vi "WriteWiringToMap.vi"(8 "error in (no error)":errorcluster, 9 "Map in":T12, 10 "Working Current":T1, 11 "Group":T2) -> (0 "error out":errorcluster, 1 "Map out":T12, 3 "Group out":T2)   [LabVIEW 2017, in "McsaAnalysisLowRate.lvlib"]
uses:
  <vilib>/addons/InsightCM/Devices/Shared/Mcsa/McsaAnalysisLowRate/McsaAnalysisLowRate.lvlib
  <vilib>/addons/PointValueMap/controls/PointMap.ctl
  <vilib>/addons/InsightCM/Devices/Shared/Mcsa/McsaAnalysisLowRate/controls/Group.ctl
  <vilib>/addons/InsightCM/Utilities/Analysis/MCSA/controls/McsaChannel.ctl
  <vilib>/addons/InsightCM/Utilities/Analysis/Shared/controls/Feature.ctl
  <vilib>/addons/InsightCM/Utilities/Analysis/Shared/controls/AmplitudeScale.ctl
  <vilib>/addons/InsightCM/MessageBus/Base/controls/KeyValuePair.ctl
  <vilib>/addons/InsightCM/Utilities/Analysis/MCSA/controls/McsaChannelPhasor.ctl
  <vilib>/addons/InsightCM/Utilities/Analysis/MCSA/controls/McsaMotor.ctl
  <vilib>/addons/InsightCM/Utilities/Analysis/MCSA/controls/MotorCalculationCache.ctl
  <vilib>/addons/Electrical Power/Basic/Measurement/subVIs/basic_Power Value.ctl
  <vilib>/addons/InsightCM/Utilities/Analysis/MCSA/controls/TorqueLoadEfficiency.ctl
  <vilib>/addons/InsightCM/Utilities/Analysis/MCSA/controls/WorkingCurrent.ctl
  <vilib>/addons/InsightCM/Utilities/MCSA/McsaUtilities.lvlib
  <vilib>/addons/PointValueMap/PointValueMap.lvlib
  <vilib>/addons/InsightCM/Utilities/Analysis/Shared/AnalysisHelper.lvlib
  <vilib>/addons/InsightCM/Utilities/Analysis/MCSA/McsaAnalysisFunctions.lvlib
  <vilib>/addons/Electrical Power/Basic/NI_EP_Basic.lvlib
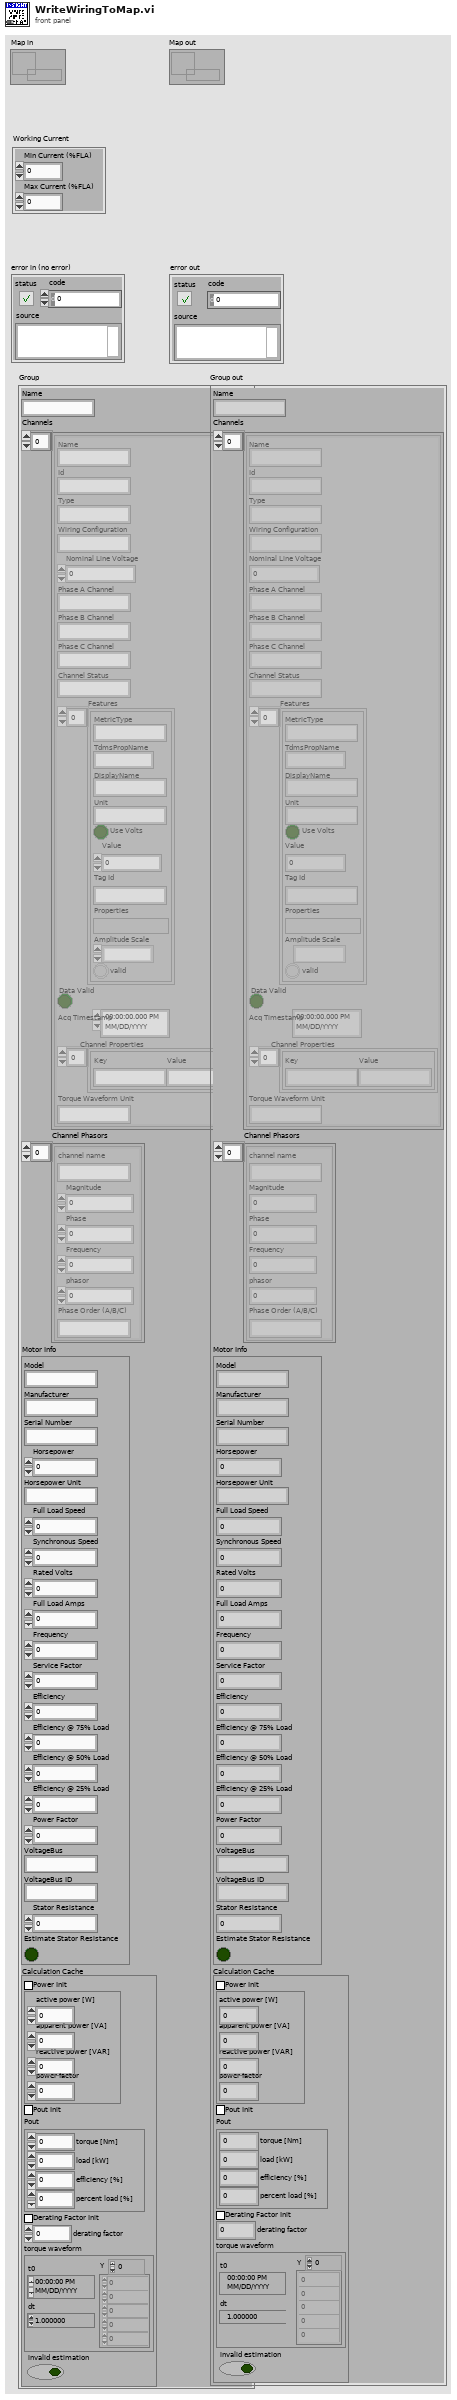
[diagram p1: front panel]
types:
  T1 = typedef "McsaAnalysisFunctions.lvlib/WorkingCurrent.ctl" = cluster{"Min Current (%FLA)":dbl, "Max Current (%FLA)":dbl}
  T2 = typedef "McsaAnalysisLowRate.lvlib/Group.ctl" = cluster{"Name":string, "Channels":T3[], "Channel Phasors":T7[], "Motor Info":T8, "Calculation Cache":T9}
  T3 = typedef "McsaAnalysisFunctions.lvlib/McsaChannel.ctl" = cluster{"Name":string, "Id":string, "Type":string, "Wiring Configuration":string, "Nominal Line Voltage":dbl, "Phase A Channel":string, "Phase B Channel":string, "Phase C Channel":string, "Channel Status":string, "Features":T4[], "Data Valid":bool, "Acq Timestamp":timestamp, "Channel Properties":T6[], "Torque Waveform Unit":string}
  T4 = typedef "AnalysisHelper.lvlib/Feature.ctl" = cluster{"MetricType":string, "TdmsPropName":string, "DisplayName":string, "Unit":string, "Use Volts":bool, "Value":dbl, "Tag Id":string, "Properties":variant, "Amplitude Scale":T5, "valid":bool}
  T5 = typedef "AnalysisHelper.lvlib/AmplitudeScale.ctl" = enum16{"rms", "peak", "pk-pk"}
  T6 = typedef "KeyValuePair.ctl" = cluster{"Key":string, "Value":string}
  T7 = typedef "McsaAnalysisFunctions.lvlib/McsaChannelPhasor.ctl" = cluster{"channel name":string, "Magnitude":dbl, "Phase":dbl, "Frequency":dbl, "phasor":cdb, "Phase Order (A/B/C)":string}
  T8 = typedef "McsaAnalysisFunctions.lvlib/McsaMotor.ctl" = cluster{"Model":string, "Manufacturer":string, "Serial Number":string, "Horsepower":dbl, "Horsepower Unit":string, "Full Load Speed":dbl, "Synchronous Speed":dbl, "Rated Volts":dbl, "Full Load Amps":dbl, "Frequency":dbl, "Service Factor":dbl, "Efficiency":dbl, "Efficiency @ 75% Load":dbl, "Efficiency @ 50% Load":dbl, "Efficiency @ 25% Load":dbl, "Power Factor":dbl, "VoltageBus":string, "VoltageBus ID":string, "Stator Resistance":dbl, "Estimate Stator Resistance":bool}
  T9 = typedef "McsaAnalysisFunctions.lvlib/MotorCalculationCache.ctl" = cluster{"Power Init":bool, "power value":T10, "Pout Init":bool, "Pout":T11, "Derating Factor Init":bool, "derating factor":sgl, "torque waveform":waveform(dbl), "invalid estimation":bool}
  T10 = typedef "NI_EP_Basic.lvlib/basic_Power Value.ctl" = cluster{"active power [W]":dbl, "apparent power [VA]":dbl, "reactive power [VAR]":dbl, "power factor":dbl}
  T11 = typedef "McsaAnalysisFunctions.lvlib/TorqueLoadEfficiency.ctl" = cluster{"torque [Nm]":dbl, "load [kW]":dbl, "efficiency [%]":dbl, "percent load [%]":dbl}
  T12 = typedef "PointValueMap.lvlib/PointMap.ctl" = refnum<data-value>
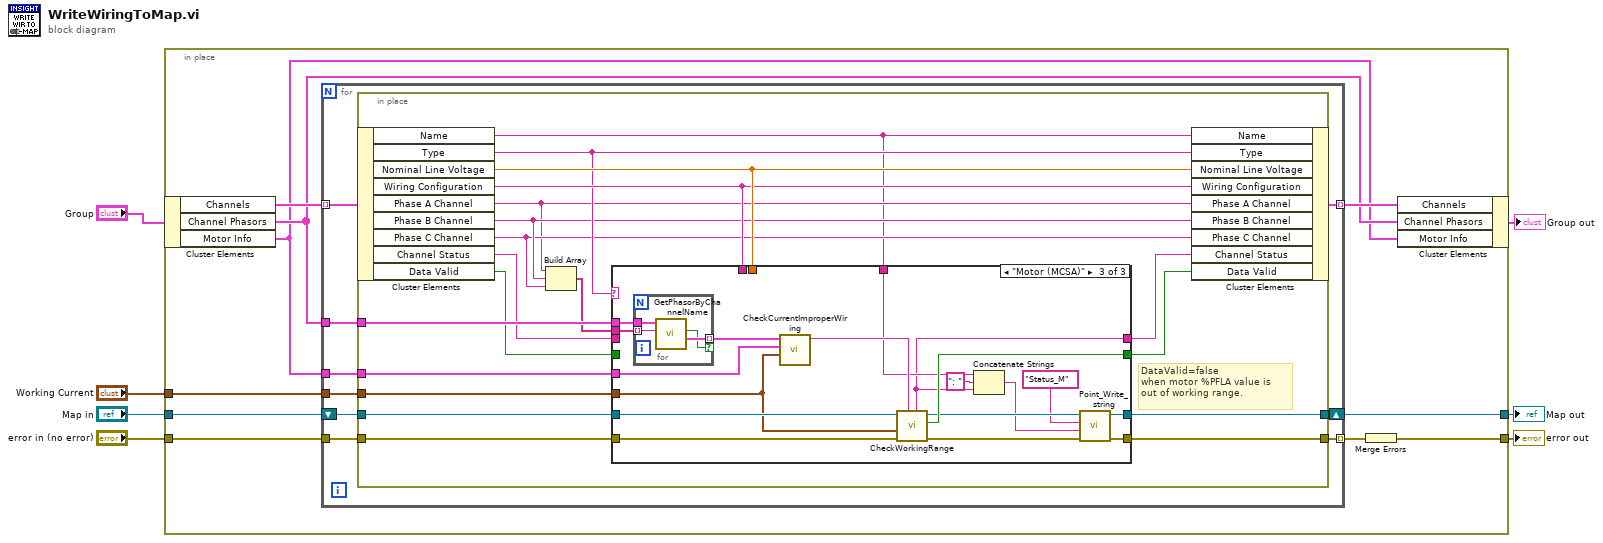
[diagram p0: block diagram]
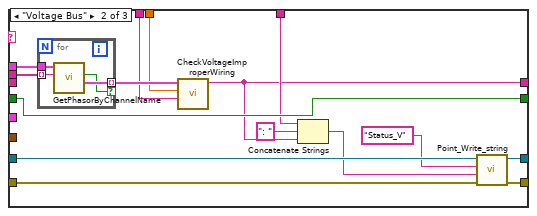
[diagram p3: hidden frame]
diagram:
  n1 = in-place {
    in-place-border: "Map in" -> [w17]
    in-place-border: "error in (no error)" -> [w16]
    in-place-border: [w10] -> w7
    in-place-border: [w9] -> w4
    in-place-border: "Working Current" -> [w11]
    n2 = in-place-cluster #1("Group") -> ("Channels"=w14:T3[], "Channel Phasors"=w12:T7[], "Motor Info"=w8:T8)
    n3 = for {
      tunnel: w14 -> [w21] mode=indexing
      tunnel: w16 -> [w25]
      tunnel: [w24] -> w15 mode=indexing
      shift-right: [w23] -> w9
      shift-left: w17 -> [w26]
      tunnel: [w22] -> w13 mode=indexing
      tunnel: w12 -> [w20]
      tunnel: w11 -> [w19]
      tunnel: w8 -> [w18]
      n4 = in-place {
        in-place-border: w26 -> [w45]
        in-place-border: w25 -> [w44]
        in-place-border: [w38] -> w24
        in-place-border: [w43] -> w23
        in-place-border: w20 -> [w42]
        in-place-border: w19 -> [w36]
        in-place-border: w18 -> [w27]
        # "DataValid=false\nwhen motor %PFLA value is \nout of working range."
        n5 = in-place-cluster #2(w21) -> ("Name"=w28:string, "Type"=w39:string, "Nominal Line Voltage"=w41:dbl, "Wiring Configuration"=w40:string, "Phase A Channel"=w29:string, "Phase B Channel"=w31:string, "Phase C Channel"=w30:string, "Channel Status"=w35:string, "Data Valid"=w32:bool)
        n6 = Build Array(w29, w31, w30) -> (w37:string[])
        n7 = case shown="\"Motor (MCSA)\"" w39 {
          tunnel: w45 -> [w47 w55 w82]
          tunnel: w44 -> [w48 w56 w83]
          tunnel: [w47 w58 w76] -> w43
          tunnel: [w48 w57 w77] -> w38
          tunnel: [w49 w52 w72] -> w34
          tunnel: w42 -> [_ w64 w86]
          tunnel: w37 -> [_ w63 w85]
          tunnel: w41 -> [_ w61 _]
          tunnel: w40 -> [_ w60 _]
          tunnel: w35 -> [w49 _ _]
          tunnel: [w46 w59 w81] -> w33
          tunnel: w36 -> [_ _ w80]
          tunnel: w32 -> [w46 w59 _]
          tunnel: w28 -> [_ w53 w74]
          tunnel: w27 -> [_ _ w69]
          frame Default {
          }
          frame "Voltage Bus" {
            n8 = for {
              tunnel: w64 -> [w68]
              tunnel: w63 -> [w67] mode=indexing
              tunnel: [w66] -> w62 mode=indexing if=w65
              n9 = call <vilib>:"GetPhasorByChannelName.vi"("Channel Name"=w67, "Channels Phasor"=w68) -> ("Channel Phasor"=w66:T7, "Found?"=w65:bool)  [unwired: 7 in, 1 out]
            }
            n10 = call <vilib>:"CheckVoltageImproperWiring.vi"("Wiring Configuration"=w60, "nominal voltage"=w61, "Group Phasors"=w62) -> ("wiring information"=w52:string)  [unwired: 7 in, 1 out]
            n11 = Concatenate Strings(w53, ": " ("string"), w52) -> (w54:string)
            n12 = call <vilib>:"Point_Write_string.vi"("Error In"=w56, "Value"=w54, "Tag"="Status_V", "Map"=w55) -> ("Error Out"=w57:errorcluster, "Map Out"=w58:T12)  [unwired: 6 in]
          }
          frame "Motor (MCSA)" {
            n13 = for {
              tunnel: w86 -> [w90]
              tunnel: w85 -> [w89] mode=indexing
              tunnel: [w88] -> w84 mode=indexing if=w87
              n14 = call <vilib>:"GetPhasorByChannelName.vi"("Channel Name"=w89, "Channels Phasor"=w90) -> ("Channel Phasor"=w88:T7, "Found?"=w87:bool)  [unwired: 7 in, 1 out]
            }
            n15 = call <vilib>:"CheckCurrentImproperWiring.vi"("Working Current"=w80, "Motor"=w69, "Group Phasors"=w84) -> ("wiring information"=w79:string)  [unwired: 7 in, 1 out]
            n16 = call <vilib>:"CheckWorkingRange.vi"("channel status in"=w79, "error in (no error)"=w83, "Working Current"=w80, "Map in"=w82) -> ("error out"=w78:errorcluster, "in range?"=w81:bool, "Map out"=w75:T12, "channel status out"=w72:string)  [unwired: 4 in]
            n17 = Concatenate Strings(w74, ": " ("string"), w72) -> (w71:string)
            n18 = call <vilib>:"Point_Write_string.vi"("Error In"=w78, "Value"=w71, "Tag"="Status_M", "Map"=w75) -> ("Error Out"=w77:errorcluster, "Map Out"=w76:T12)  [unwired: 6 in]
          }
        }
        n19 = in-place-cluster #2("Name"=w28, "Type"=w39, "Nominal Line Voltage"=w41, "Wiring Configuration"=w40, "Phase A Channel"=w29, "Phase B Channel"=w31, "Phase C Channel"=w30, "Channel Status"=w34, "Data Valid"=w33) -> (w22:T3)
      }
    }
    n20 = Merge Errors(w15) -> (w10:errorcluster)
    n21 = in-place-cluster #1("Channels"=w13, "Channel Phasors"=w12, "Motor Info"=w8) -> (→"Group out":T2)
  }
  "error out" <- w7
  "Map out" <- w4
